vi "PicoScope5000aExampleRapidBlockBulk.vi"() -> ()   [LabVIEW 2009]
panel:
  in  "Serial Number":string
  in  "Use Serial Number":bool
  out "Number of Samples \nPer Capture":u32
  in  "Resolution":i32(ring) items=["8-bit", "12-bit", "14-bit", "15-bit (max. 2 ch.)", "16-bit (max. 1 ch.)"]
  in  "PS5X4XA/B\nUSB Powered":bool
  in  "Trigger Settings":T1 {"Trigger Direction" items=["Rising", "Falling"]}
  in  "Channel A Settings":T2 {"Range" items=["10 mV", "20 mV", "50 mV", "100 mV", "200 mV", "500 mV", "1 V", "2 V", "5 V", "10 V", "20 V", "50 V ", "100 V"]; "Coupling" items=["AC", "DC"]}
  in  "Rapid Block Acquisition Settings":T3
  out "Capture Complete":bool
  in  "Run":bool
  out "Channel A":i16[](graph)
  in  "Capture Index":i16 min=0
  in  "stop":bool
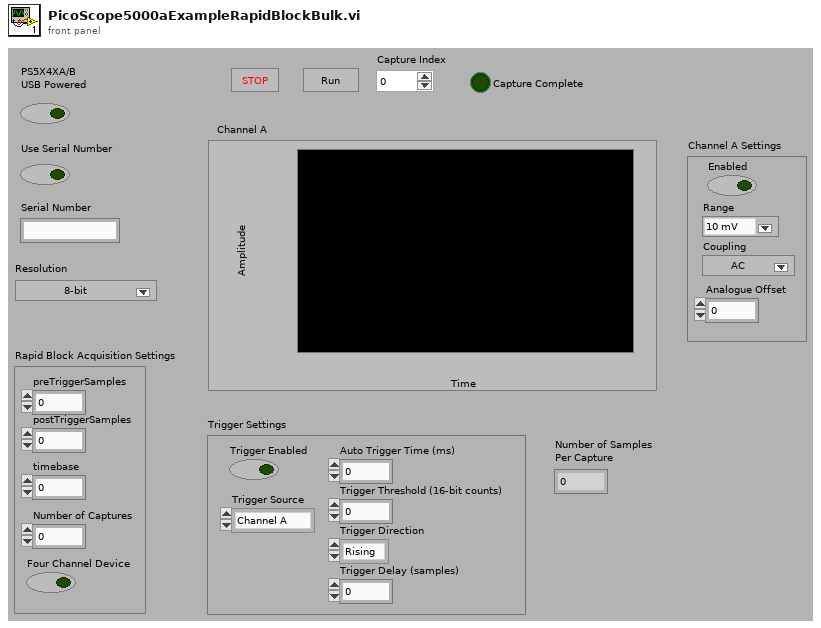
[diagram p1: front panel]
types:
  T1 = cluster{"Trigger Enabled":bool, "Trigger Source":enum16{"Channel A", "Channel B", "Channel C", "Channel D", "Ext."}, "Trigger Threshold (16-bit counts)":i16, "Trigger Direction":u16, "Trigger Delay (samples)":u32, "Auto Trigger Time (ms)":i16}
  T2 = cluster{"Enabled":bool, "Coupling":i16, "Range":u16, "Analogue Offset":sgl}
  T3 = cluster{"preTriggerSamples":u32, "postTriggerSamples":u32, "timebase":u32, "Four Channel Device":bool, "Number of Captures":u32}
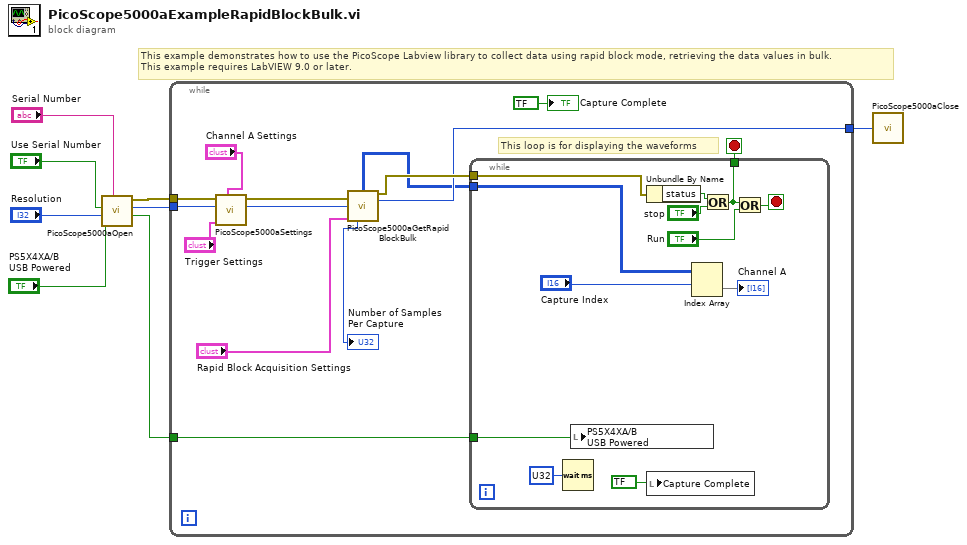
[diagram p0: block diagram]
diagram:
  # "This example demonstrates how to use the PicoScope Labview library to collect data using rapid block mode, retrieving the data values in bulk.\nThis example requires LabVIEW 9.0 or later."
  n1 = call "PicoScope5000aOpen.vi"("Serial Number"="Serial Number", "USB Powered Selection"="PS5X4XA/B\nUSB Powered", "Resolution"="Resolution", "Use Serial Number"="Use Serial Number") -> ("USB Powered Indication"=w4:bool, "handle"=w6:i16, "error out"=w7:errorcluster)  [unwired: 3 in, 2 out]
  n2 = while {
    tunnel: [w18] -> w8
    tunnel: w7 -> [w13]
    tunnel: w6 -> [w12]
    tunnel: w4 -> [w11]
    stop <- w22 stop-if-true
    # "This loop is for displaying the waveforms"
    n3 = call "PicoScope5000aSettings.vi"("Channel A Settings"="Channel A Settings", "Trigger Settings"="Trigger Settings", "handle in"=w12, "error in"=w13) -> ("handle out"=w17:i16, "error out"=w16:errorcluster)  [unwired: 6 in]
    n4 = call "PicoScope5000aGetRapidBlockBulk.vi"("error in"=w16, "handle in"=w17, "Rapid Block Acquisition Settings"="Rapid Block Acquisition Settings") -> ("Channel A Buffer"=w9:i16[][], "error out"=w19:errorcluster, "handle out"=w18:i16, "Num samples"=→"Number of Samples \nPer Capture":u32)  [unwired: 6 in, 3 out]
    n5 = while {
      tunnel: [w33] -> w22
      tunnel: w9 -> [w25]
      tunnel: w19 -> [w28]
      tunnel: w11 -> [w26]
      stop <- w32 stop-if-true
      n6 = Wait (ms)(milliseconds to wait=u32 ?) -> ()  [unwired: 1 out]
      n7 = local write "PS5X4XA/B\nUSB Powered"(w26) -> ()
      n8 = Unbundle By Name(w28) -> ("status"=w27:bool)
      n9 = local write "Capture Complete"(bool ? ("Capture Complete")) -> ()
      n10 = Index Array(array=w25, index (row)="Capture Index") -> (element=→"Channel A":i16[])  [unwired: 1 in]
      n11 = Or(x=w27, y="stop") -> (x .or. y?=w33:bool)
      n12 = Or(x=w33, y="Run") -> (x .or. y?=w32:bool)
    }
    "Capture Complete" <- bool ? ("Capture Complete")
  }
  n13 = call "PicoScope5000aClose.vi"("handle"=w8) -> ()
